vi "InitScanner.vi"(8 "error in (no error)":errorcluster, 11 "PI SystemNumber":i32) -> (0 "error out":errorcluster, 1 "z-position":dbl, 2 "y-position":dbl, 3 "x-position":dbl, 5 "Conn. Axes":string[](array[string]))   [LabVIEW 2011]
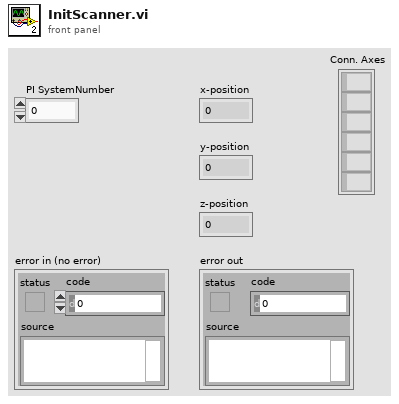
[diagram p1: front panel]
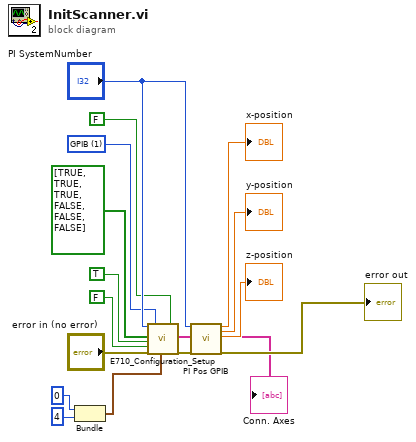
[diagram p0: block diagram]
diagram:
  w11 = u16 1 items=["RS232", "GPIB"] ("Interface")
  n1 = Bundle(0, 4) -> (w13:cluster{i32, i32})  [unwired: 1 out]
  n2 = call "E710_Configuration_Setup.vi"("System no."="PI SystemNumber", "Are stages connected?"=bool[] [TRUE, TRUE, TRUE, FALSE, FALSE, FALSE], "Change servo \nstatus to ON?"=TRUE ("Change servo \nstatus to ON?"), "Perform autozero?"=FALSE ("All axes?"), "error in"="error in (no error)", "Interface"=w11, "GPIB settings"=w13, "Move to middle?"=FALSE) -> ("Conn. Axes"=→"Conn. Axes":string[], "error out"=w2:errorcluster)  [unwired: 4 in, 6 out]
  n3 = call "PI Pos GPIB.vi"("System no."="PI SystemNumber", "error in"=w2) -> ("x-position"=→"x-position":dbl, "y-position"=→"y-position":dbl, "z-position"=→"z-position":dbl, "error out"=→"error out":errorcluster)  [unwired: 14 in]
